vi "AlliGator Phasor Ratio Reference String.vi"(8 "error in (no error)":errorcluster, 11 "Reference #":i32) -> (0 "Error Out":errorcluster, 3 "Message":string)   [LabVIEW 2021, in "AlliGator Phasor Ratio.lvlib"]
doc: "Builds phasor reference output string."
uses:
  AlliGator Phasor Ratio.lvlib
  Phasor/Phasor.lvlib
panel:
  # "see the AlliGator License on the block diagram (Ctrl+E or Window:Show Block Diagram)"
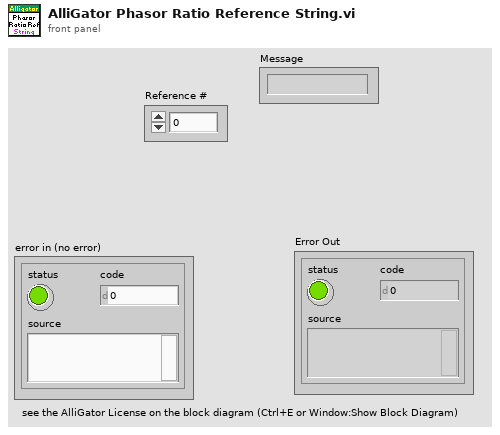
[diagram p1: front panel]
types:
  T1 = typedef "Phasor.lvlib/Phasor (g, s).ctl" = cluster{"g":dbl, "s":dbl}
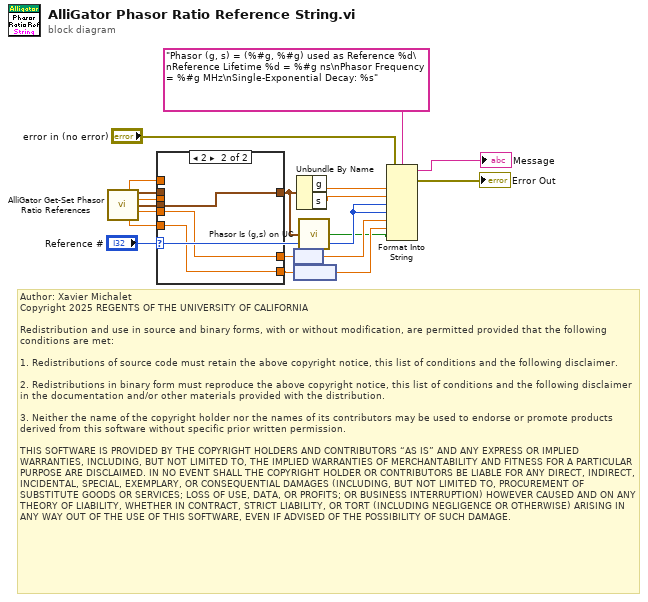
[diagram p0: block diagram]
diagram:
  # "Author: Xavier Michalet\nCopyright 2025 REGENTS OF THE UNIVERSITY OF CALIFORNIA\n\nRedistribution and use in source and binary forms, with or without modification, are permitted provided that the following conditions are met:\n\n1. Redistributions of source code must retain the above copyright notice, this list of conditions and the following disclaimer.\n\n2. Redistributions in binary form must reproduce the above copyright notice, this list of conditions and the following disclaimer in the documentation and/or other materials provided with the distribution.\n\n3. Neither the name of the copyright holder nor the names of its contributors may be used to endorse or promote products derived from this software without specific prior written permission.\n\nTHIS SOFTWARE IS PROVIDED BY THE COPYRIGHT HOLDERS AND CONTRIBUTORS “AS IS” AND ANY EXPRESS OR IMPLIED WARRANTIES, INCLUDING, BUT NOT LIMITED TO, THE IMPLIED WARRANTIES OF MERCHANTABILITY AND FITNESS FOR A PARTICULAR PURPOSE ARE DISCLAIMED. IN NO EVENT SHALL THE COPYRIGHT HOLDER OR CONTRIBUTORS BE LIABLE FOR ANY DIRECT, INDIRECT, INCIDENTAL, SPECIAL, EXEMPLARY, OR CONSEQUENTIAL DAMAGES (INCLUDING, BUT NOT LIMITED TO, PROCUREMENT OF SUBSTITUTE GOODS OR SERVICES; LOSS OF USE, DATA, OR PROFITS; OR BUSINESS INTERRUPTION) HOWEVER CAUSED AND ON ANY THEORY OF LIABILITY, WHETHER IN CONTRACT, STRICT LIABILITY, OR TORT (INCLUDING NEGLIGENCE OR OTHERWISE) ARISING IN ANY WAY OUT OF THE USE OF THIS SOFTWARE, EVEN IF ADVISED OF THE POSSIBILITY OF SUCH DAMAGE."
  n1 = call "AlliGator Get-Set Phasor Ratio References.vi"() -> ("Reference Frequency 1"=w5:dbl[unit], "Reference Phasor 1"=w13:T1, "Reference Lifetime 1"=w11:dbl[unit], "Reference Phasor 2"=w10:T1, "Reference Lifetime 2"=w9:dbl[unit], "Reference Frequency 2"=w6:dbl[unit])  [unwired: 8 in, 2 out]
  n2 = case shown="2" "Reference #" {
    tunnel: w13 -> [w22 _]
    tunnel: [w22 w23] -> w2
    tunnel: [w21 w25] -> w12
    tunnel: w11 -> [w21 _]
    tunnel: w10 -> [_ w23]
    tunnel: w9 -> [_ w25]
    tunnel: w6 -> [_ w24]
    tunnel: w5 -> [w20 _]
    tunnel: [w20 w24] -> w4
    frame 1, Default {
    }
    frame 2 {
    }
  }
  n3 = node(w12) -> (w15:dbl)
  n4 = node(w4) -> (w3:dbl)
  n5 = Unbundle By Name(w2) -> ("g"=w8:dbl, "s"=w7:dbl)
  n6 = call "Phasor Is (g,s) on UC.vi"("Phasor (g, s)"=w2) -> ("Is on UC?"=w1:bool)  [unwired: 8 in]
  n7 = Format Into String(format string="Phasor (g, s) = (%#g, %#g) used as Reference %d\nReference Lifetime %d = %#g ns\nPhasor Frequency = %#g MHz\nSingle-Exponential Decay: %s", error in="error in (no error)", w8, w7, "Reference #", "Reference #", w15, w3, w1) -> (resulting string=→"Message":string, error out=→"Error Out":errorcluster)  [unwired: 1 in]
